vi "ErrorHandlerFunctionalGlobal.vi"(8 "error in (no error)":errorcluster, 11 "Command Input":T1) -> (0 "single error out":errorcluster, 1 "Collection of Errors Output":errorcluster[](array[cluster]))   [LabVIEW 2016]
doc: "Overview: This example demonstrates an architecture for a subVI that can be called throughout an application to collect all possible errors that have occurred and report them in a list, in the form of an Array Indicator.\n\nSelect one of the following commands in the Command Input to perform different tasks:\n a) Initialize: This state assigns an empty array of errors to the FGV. Use to reinitialize the internal error array. \n b) Handle Errors: Default state, it saves any errors coming in to the internal error array.\n c) Report Errors: This State should be called at the end to see all error as and array output."
uses:
  Error Handler Command Input.ctl
panel:
  # "Multiple Error Handling FGV\n\nOverview: This example demonstrates an architecture for a subVI that can be called throughout an application to\ncollect all possible errors that have occurred and report them in a list, in the form of an Array Indicator.\nRequirements: NI LabVIEW Base Development System 2012 (or compatible).\nInstructions: \n1. Call this VI from another VI, since this is an FGV (Functional Global Variable).\n2. Select one of the following commands in the Command Input to perform different tasks:\n    a) Initialize: This state assigns an empty array of errors to the FGV. Use to reinitialize the internal error array. \n    b) Handle Errors: Default state, it saves any errors coming in to the internal error array.\n    c) Report Errors: This State should be called at the end to see all error as and array output."
  # "Input Data"
  # "Output Data"
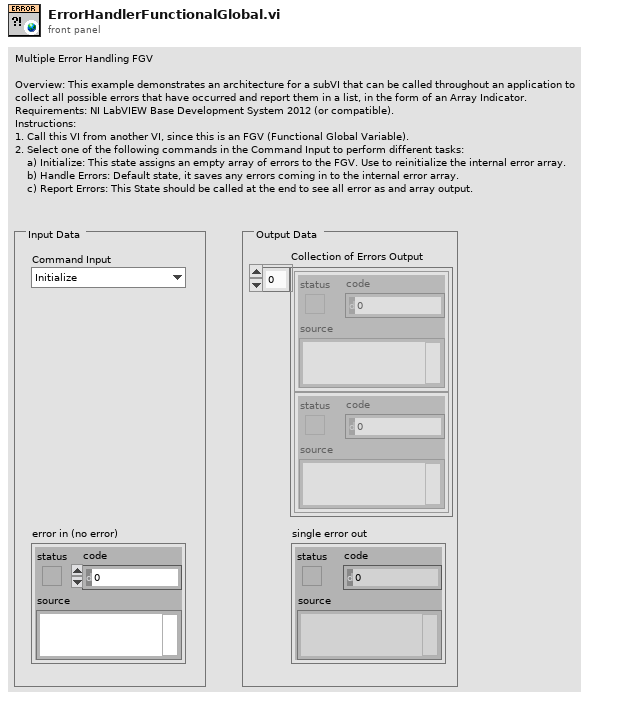
[diagram p1: front panel]
types:
  T1 = typedef "Error Handler Command Input.ctl" = enum16{"Initialize", "Handle Errors", "Report Errors"}
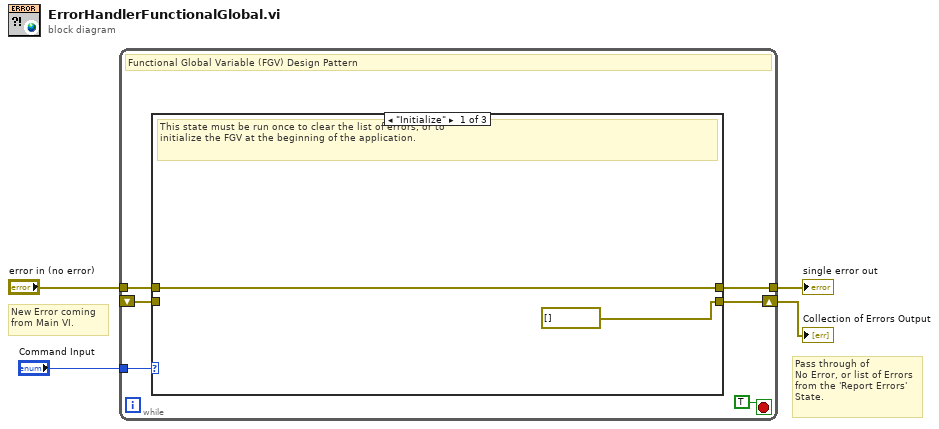
[diagram p0: block diagram]
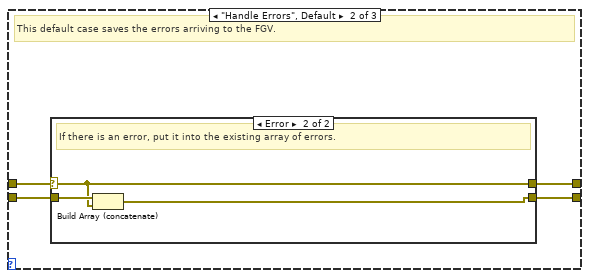
[diagram p2: hidden frame]
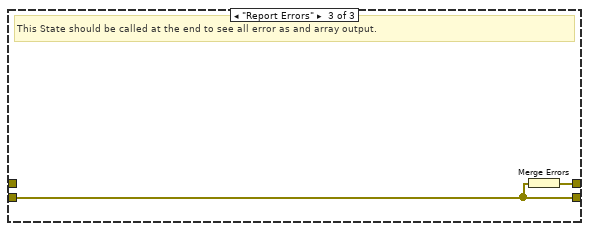
[diagram p4: hidden frame]
diagram:
  # "Pass through of\nNo Error, or list of Errors\nfrom the 'Report Errors'\nState."
  # "New Error coming\nfrom Main VI."
  n1 = while {
    tunnel: "error in (no error)" -> [w9]
    tunnel: [w8] -> w3
    shift-right: [w6] -> w1
    shift-left: _ -> [w7]
    tunnel: "Command Input" -> [w5]
    stop <- TRUE stop-if-true
    # "Functional Global Variable (FGV) Design Pattern"
    n2 = case shown="\"Initialize\"" w5 {
      tunnel: w9 -> [w11 w16 _]
      tunnel: [w11 w15 w23] -> w8
      tunnel: w7 -> [_ w14 w22]
      tunnel: [errorcluster[] [] ("Collection of Errors") w13 w22] -> w6
      frame "Initialize" {
        # "This state must be run once to clear the list of errors, or to \ninitialize the FGV at the beginning of the application."
      }
      frame "Handle Errors", Default {
        # "This default case saves the errors arriving to the FGV."
        n3 = case shown="Error" w16 {
          selector: w16 -> [w18 w19]
          tunnel: [w18 w19] -> w15
          tunnel: w14 -> [w17 w21]
          tunnel: [w17 w20] -> w13
          frame No Error {
            # "If there is No Error, don't do anything."
          }
          frame Error {
            # "If there is an error, put it into the existing array of errors."
            n4 = Build Array (concatenate)(w21, w19) -> (w20:errorcluster[])
          }
        }
      }
      frame "Report Errors" {
        # "This State should be called at the end to see all error as and array output."
        n5 = Merge Errors(w22) -> (w23:errorcluster)
      }
    }
  }
  "single error out" <- w3
  "Collection of Errors Output" <- w1
